vi "Skip_If Sd_Error_Below.vi"(0 "String to Search":string, 1 "Simulate/Run":T1, 2 "Measurement setup Applied?":bool, 3 "Row Number":i32, 5 "Measurement Setup File":string) -> (4 "Check for Skip?":bool, 6 "Error String":string, 7 "Instrument Code Name":string, 8 "Sd Error Theshold value":dbl, 9 "Minimum Measurement time (Sec)":dbl=6.0 format="%.2f")   [LabVIEW 2010]
uses:
  Controls/User_Specific_mode.ctl
  Globals/Extra_Commands_Global.vi
  Globals/Meas_global.vi
  Globals/Constants_global.vi
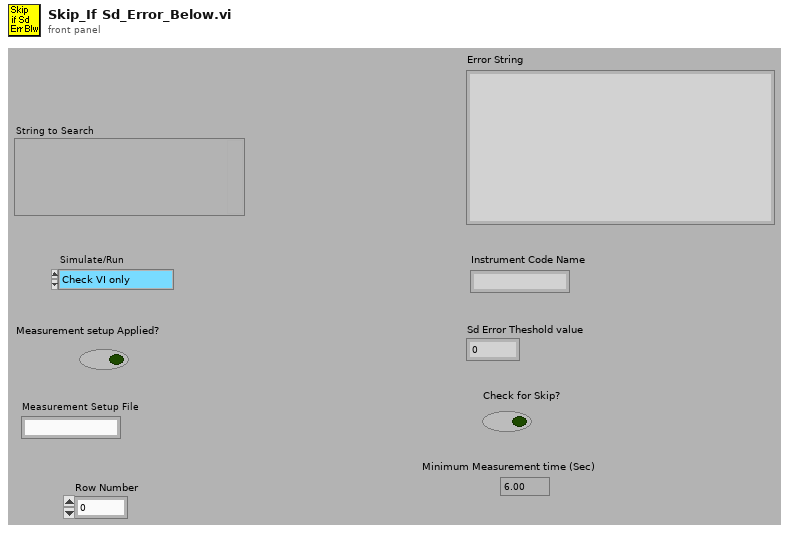
[diagram p1: front panel]
types:
  T1 = typedef "User_Specific_mode.ctl" = enum16{"Check VI only", "Run VI"}
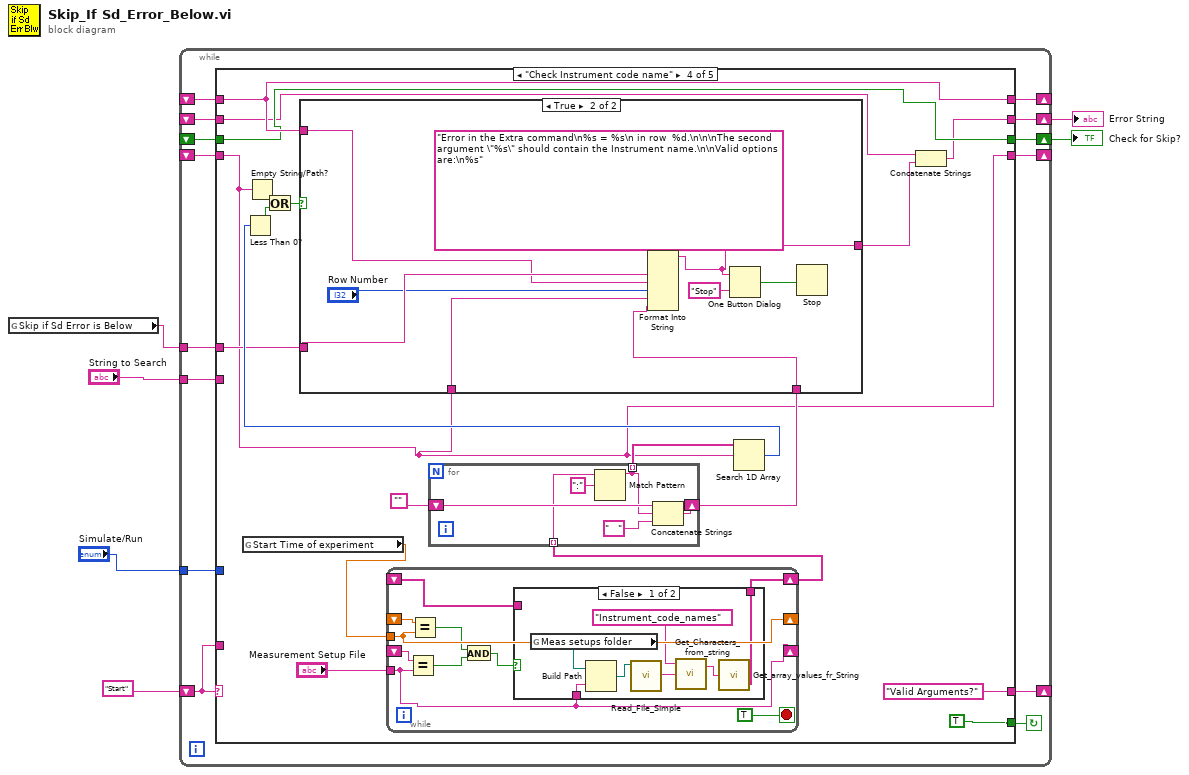
[diagram p0: block diagram]
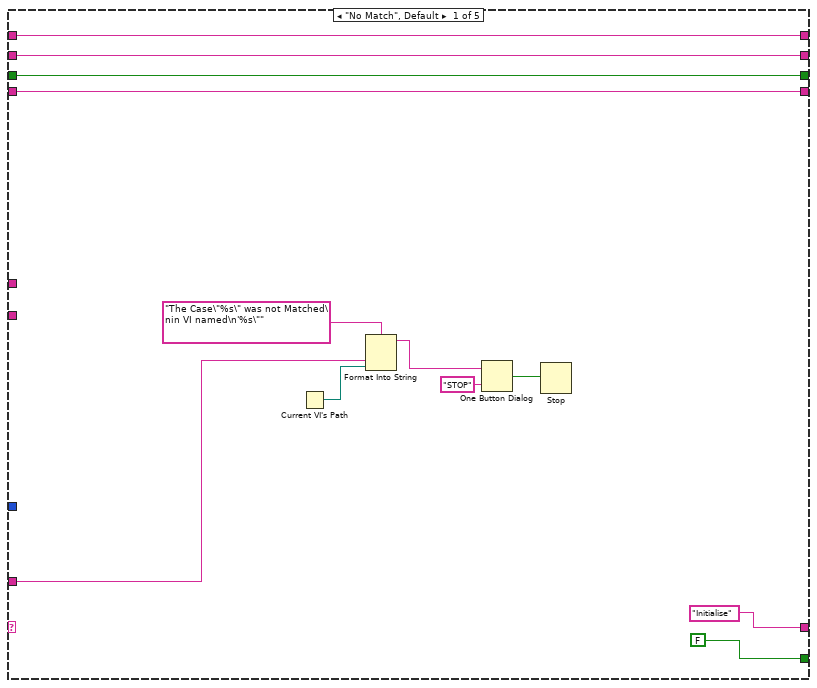
[diagram p2: hidden frame]
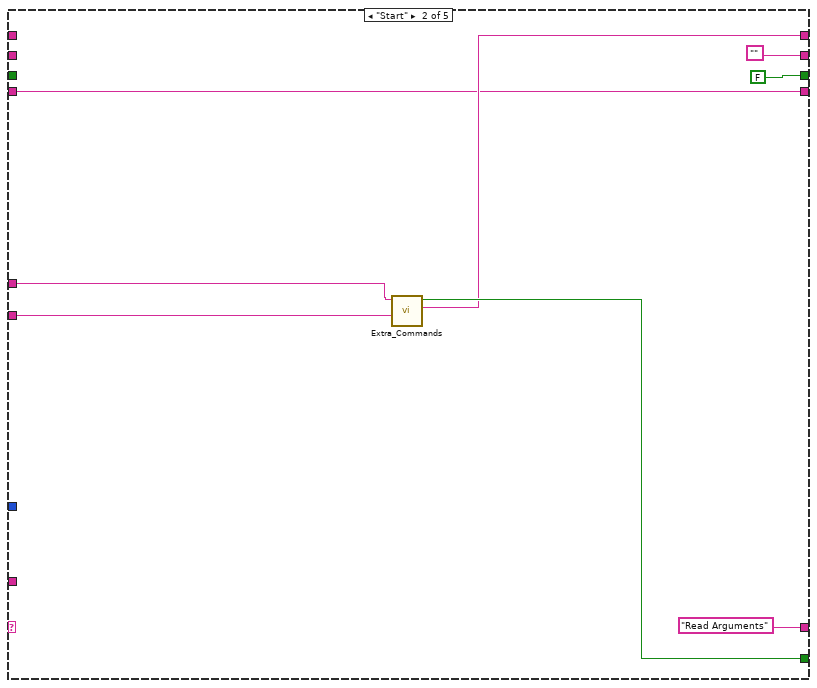
[diagram p3: hidden frame]
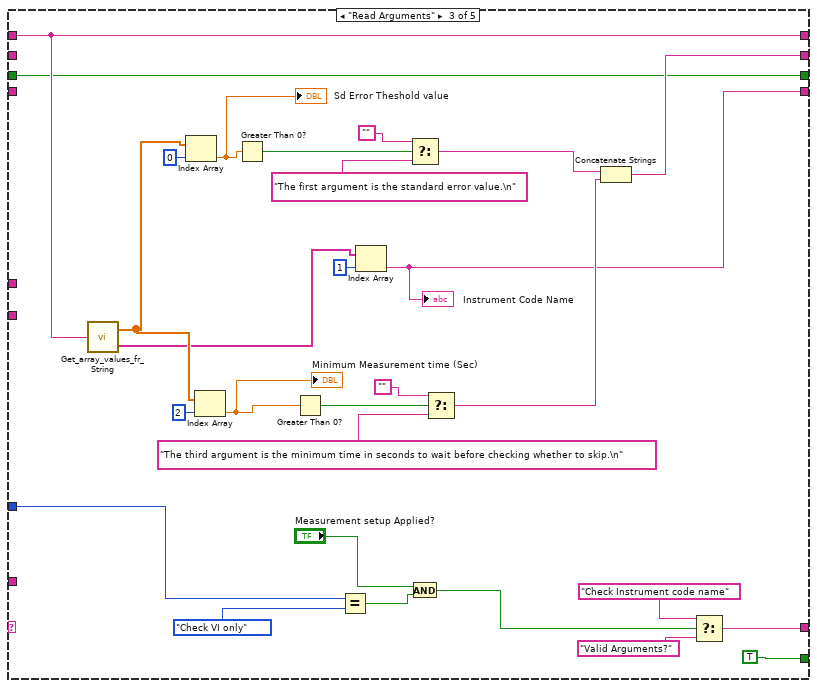
[diagram p4: hidden frame]
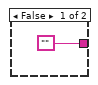
[diagram p6: hidden frame]
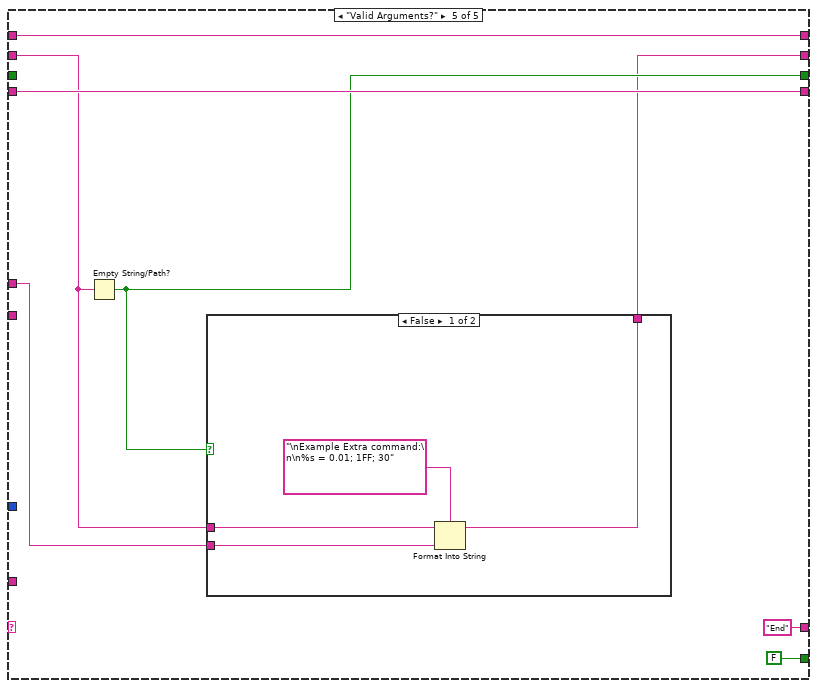
[diagram p7: hidden frame]
diagram:
  n1 = global read "Extra_Commands_Global.vi" "Skip if Sd Error is Below"() -> (w2:string)
  n2 = while {
    shift-left: "Start" -> [w18]
    shift-right: [w19] -> _
    tunnel: "String to Search" -> [w17]
    shift-right: [w16] -> _
    shift-left: _ -> [w13]
    shift-right: [w14] -> w4
    shift-left: _ -> [w12]
    shift-right: [w15] -> w3
    shift-left: _ -> [w11]
    tunnel: w2 -> [w10]
    shift-right: [w8] -> _
    shift-left: _ -> [w9]
    tunnel: "Simulate/Run" -> [w7]
    stop <- w20 continue-if-true
    n3 = case shown="\"Check Instrument code name\"" w18 {
      tunnel: [FALSE w38 TRUE TRUE FALSE ("Command Found")] -> w20
      tunnel: ["Initialise" "Read Arguments" w54 "Valid Arguments?" "End"] -> w19
      tunnel: w18 -> [w27 _ _ _ _]
      tunnel: w17 -> [_ w39 _ _ _]
      tunnel: [w24 w37 w52 w81 w129] -> w16
      tunnel: [w22 FALSE w45 w80 w125] -> w15
      tunnel: [w23 "" w46 w76 w122] -> w14
      tunnel: w13 -> [w24 _ w52 w81 w129]
      tunnel: w12 -> [w23 _ _ w78 w123]
      tunnel: w11 -> [w22 _ w45 w80 _]
      tunnel: w10 -> [_ w34 _ w82 w124]
      tunnel: w9 -> [w21 w33 _ w73 w128]
      tunnel: [w21 w33 w42 w73 w128] -> w8
      tunnel: w7 -> [_ _ w50 _ _]
      frame "No Match", Default {
        n4 = Current VI's Path() -> (path=w26:path)
        n5 = Format Into String(format string="The Case\"%s\" was not Matched\nin VI named\n'%s\"" ("Format String"), w27, w26) -> (resulting string=w30:string)  [unwired: 2 in, 1 out]
        n6 = One Button Dialog(message=w30, button name ("OK")="STOP") -> (true=w28:bool)
        n7 = Stop(stop? (T)=w28) -> ()
      }
      frame "Start" {
        n8 = call "Extra_Commands.vi"("String to Search"=w39, "Command"=w34) -> ("String Value"=w37:string, "Command Found"=w38:bool)  [unwired: 1 in, 3 out]
      }
      frame "Read Arguments" {
        n9 = call "Get_array_values_fr_String.vi"("String Value"=w52) -> ("Numeric Array"=w61:dbl[], "String array"=w57:string[])
        n10 = Index Array(array=w61, index=0) -> (element=w43:dbl)
        "Sd Error Theshold value" <- w43
        n11 = Index Array(array=w61, index=2) -> (element=w44:dbl)
        "Minimum Measurement time (Sec)" <- w44
        n12 = Greater Than 0?(x=w43) -> (x > 0?=w64:bool)
        n13 = Greater Than 0?(x=w44) -> (x > 0?=w58:bool)
        n14 = Equal?(x=w50, y=User_Specific_mode."Check VI only" ("Simulate/Run")) -> (x = y?=w49:bool)
        n15 = Index Array(array=w57, index=1) -> (element=w42:string)
        "Instrument Code Name" <- w42
        n16 = Select(t="", s=w64, f="The first argument is the standard error value.\n") -> (s? t:f=w56:string)
        n17 = And(x="Measurement setup Applied?", y=w49) -> (x .and. y?=w47:bool)
        n18 = Select(t="", s=w58, f="The third argument is the minimum time in seconds to wait before checking whether to skip.\n") -> (s? t:f=w55:string)
        n19 = Concatenate Strings(w56, w55) -> (w46:string)
        n20 = Select(t="Check Instrument code name", s=w47, f="Valid Arguments?") -> (s? t:f=w54:string)
      }
      frame "Check Instrument code name" {
        n21 = global read "Meas_global.vi" "Start Time of experiment"() -> (w69:dbl)
        n22 = Empty String/Path?(string/path=w73) -> (empty?=w74:bool)
        n23 = while {
          shift-right: [w96] -> w70
          shift-left: _ -> [w95]
          shift-right: [w93] -> _
          shift-left: _ -> [w97]
          tunnel: "Measurement Setup File" -> [w93]
          shift-right: [w91] -> _
          shift-left: _ -> [w92]
          tunnel: w69 -> [w91]
          stop <- TRUE stop-if-true
          n24 = Equal?(x=w97, y=w93) -> (x = y?=w89:bool)
          n25 = Equal?(x=w92, y=w91) -> (x = y?=w90:bool)
          n26 = And(x=w90, y=w89) -> (x .and. y?=w88:bool)
          n27 = case shown="False" w88 {
            tunnel: [w99 w105] -> w96
            tunnel: w95 -> [_ w105]
            tunnel: w93 -> [w98 _]
            frame False {
              n28 = global read "Constants_global.vi" "Meas setups folder"() -> (w104:path)
              n29 = Build Path(base path=w104, name or relative path=w98) -> (appended path=w101:path)
              n30 = call "Read_File_Simple.vi"("Filename"=w101) -> ("string"=w100:string)  [unwired: 2 in, 7 out]
              n31 = call "Get_Characters_from_string.vi"("Input string"=w100, "Variable name"="Instrument_code_names" ("Label for characters")) -> ("Value"=w102:string)  [unwired: 1 in, 1 out]
              n32 = call "Get_array_values_fr_String.vi"("String Value"=w102) -> ("String array"=w99:string[])  [unwired: 1 out]
            }
            frame True {
            }
          }
        }
        n33 = for {
          tunnel: [w119] -> w86 mode=indexing
          shift-right: [w118] -> w83
          shift-left: "" -> [w120]
          tunnel: w70 -> [w116] mode=indexing
          n34 = Match Pattern(string=w116, regular expression=":") -> (before substring=w119:string)  [unwired: 4 out]
          n35 = Concatenate Strings(w120, w119, "   " ("string")) -> (w118:string)
        }
        n36 = Search 1D Array(1D array=w86, element=w73) -> (index of element=w84:i32)  [unwired: 1 out]
        n37 = Less Than 0?(x=w84) -> (x < 0?=w75:bool)
        n38 = Or(x=w74, y=w75) -> (x .or. y?=w72:bool)
        n39 = case shown="True" w72 {
          tunnel: w83 -> [_ w112]
          tunnel: w82 -> [_ w114]
          tunnel: w81 -> [_ w107]
          tunnel: w73 -> [_ w113]
          tunnel: ["" w109] -> w77
          frame False {
          }
          frame True {
            n40 = Format Into String(format string="Error in the Extra command\n%s = %s\n in row  %d.\n\n\nThe second argument \"%s\" should contain the Instrument name.\n\nValid options are:\n%s" ("f"), w114, w107, "Row Number", w113, w112) -> (resulting string=w109:string)  [unwired: 2 in, 1 out]
            n41 = One Button Dialog(message=w109, button name ("OK")="Stop") -> (true=w110:bool)
            n42 = Stop(stop? (T)=w110) -> ()
          }
        }
        n43 = Concatenate Strings(w78, w77) -> (w76:string)
      }
      frame "Valid Arguments?" {
        n44 = Empty String/Path?(string/path=w123) -> (empty?=w125:bool)
        n45 = case shown="False" w125 {
          tunnel: w124 -> [w132 _]
          tunnel: w123 -> [w131 w134]
          tunnel: [w130 w134] -> w122
          frame False {
            n46 = Format Into String(format string="\nExample Extra command:\n\n%s = 0.01; 1FF; 30", initial string=w131, w132) -> (resulting string=w130:string)  [unwired: 1 in, 1 out]
          }
          frame True {
          }
        }
      }
    }
  }
  "Error String" <- w4
  "Check for Skip?" <- w3
